vi "2d array to distribution.vi"(4 "length":i32, 5 "start":i32, 6 "y bin":i32=100, 7 "x row":i32, 8 "error in (no error)":errorcluster, 9 "all rows":dbl[][](array[numeric]), 10 "y row":i32, 11 "x bin":i32=100) -> (0 "error out":errorcluster, 2 "Cluster":T1, 3 "Array":dbl[][](array[numeric]))   [LabVIEW 2021]
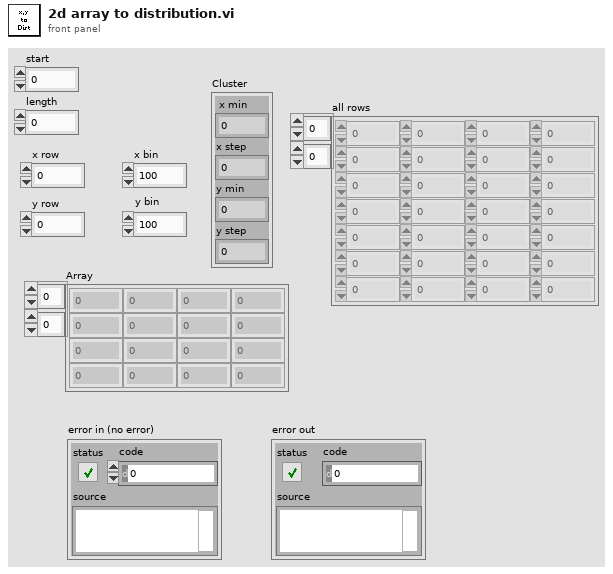
[diagram p1: front panel]
types:
  T1 = cluster{" x min":dbl, "x step":dbl, "y min":dbl, "y step":dbl}
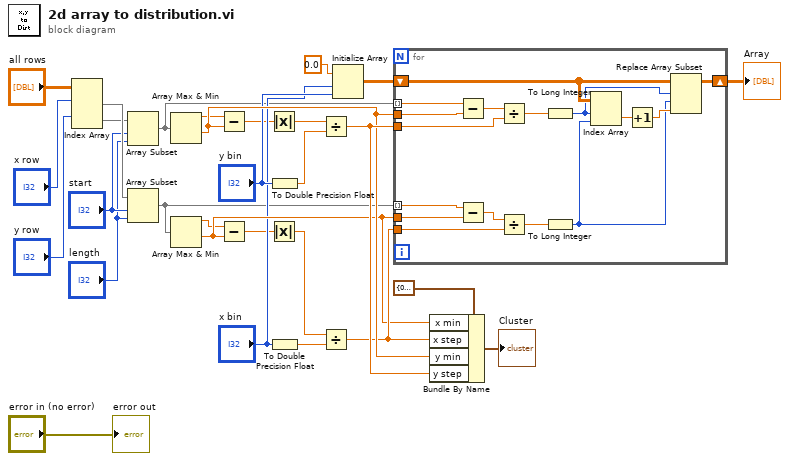
[diagram p0: block diagram]
diagram:
  n1 = Index Array(array="all rows", index (row) #1="x row", index (row) #2="y row") -> (element #1=w6:dbl[], element #2=w4:dbl[])  [unwired: 2 in]
  n2 = Array Subset(array=w4, index="start", length="length") -> (w3:dbl[])
  n3 = Array Subset(array=w6, index="start", length="length") -> (w5:dbl[])
  n4 = Array Max & Min(array=w3) -> (max value=w18:dbl, min value=w28:dbl)  [unwired: 2 out]
  n5 = Array Max & Min(array=w5) -> (max value=w11:dbl, min value=w26:dbl)  [unwired: 2 out]
  n6 = Subtract(x=w18, y=w28) -> (x-y=w15:dbl)
  n7 = Subtract(x=w11, y=w26) -> (x-y=w12:dbl)
  n8 = Absolute Value(x=w15) -> (abs(x)=w16:dbl)
  n9 = Absolute Value(x=w12) -> (abs(x)=w13:dbl)
  n10 = To Double Precision Float(number="y bin") -> (double precision float=w17:dbl)
  n11 = To Double Precision Float(number="x bin") -> (double precision float=w14:dbl)
  n12 = Divide(x=w16, y=w17) -> (x/y=w29:dbl)
  n13 = Divide(x=w13, y=w14) -> (x/y=w27:dbl)
  n14 = Initialize Array(0.0 ("element"), "x bin", "y bin") -> (w20:dbl[][])
  n15 = for {
    tunnel: w5 -> [w45] mode=indexing
    tunnel: w3 -> [w40] mode=indexing
    tunnel: w26 -> [w44]
    tunnel: w27 -> [w42]
    tunnel: w28 -> [w39]
    tunnel: w29 -> [w37]
    shift-right: [w30] -> w25
    shift-left: w20 -> [w34]
    n16 = Subtract(x=w40, y=w39) -> (x-y=w38:dbl)
    n17 = Subtract(x=w45, y=w44) -> (x-y=w43:dbl)
    n18 = Divide(x=w38, y=w37) -> (x/y=w36:dbl)
    n19 = Divide(x=w43, y=w42) -> (x/y=w41:dbl)
    n20 = To Long Integer(number=w36) -> (32bit integer=w32:i32)
    n21 = To Long Integer(number=w41) -> (32bit integer=w31:i32)
    n22 = Index Array(array=w34, index (row)=w32, index (col)=w31) -> (element=w35:dbl)
    n23 = Increment(x=w35) -> (x+1=w33:dbl)
    n24 = Replace Array Subset(array=w34, new element=w33, index (row)=w32, index (col)=w31) -> (w30:dbl[][])
  }
  "Array" <- w25
  n25 = Bundle By Name(cluster=T1 {" x min"=0.0, "x step"=0.0, "y min"=0.0, "y step"=0.0} ("Cluster"), "x min"=w26, "x step"=w27, "y min"=w28, "y step"=w29) -> (→"Cluster":T1)
  "error out" <- "error in (no error)"
